vi "Main.vi"() -> ()   [LabVIEW 2019]
doc: "This template is for the Queued Message Handler design pattern.\n\nThe Event Handling Loop generates messages based on user interface actions.\n\nThe Message Handling Loop processes messages generated by the Event Handling Loop, or by other messages. The messages are string values, so new messages can be added easily to the Message Cases case structure in the Message Handling Loop. Each message cluster can also provide an optional value for Message Data, which is a variant that can be converted to whatever message-specific data is required."
uses:
  controls/UI Data.ctl
  controls/wavedump Data.ctl
  support/Message Queue/Enqueue Message (Single).vi
  <vilib>/Utility/error.llb/Error Cluster From Error Code.vi
  <vilib>/ErrorRing/Error Ring.xnode
  support/Message Queue/Message Queue.lvlib
  support/User Event - Stop/User Event - Stop.lvlib
panel:
  in  "power":bool
  in  "Off":bool
  in  "Tab Control":enum32{"Control", "Wavedump Output", "README"}(tab)
  in  "Gain":bool
  in  "HV Channel":string[](array[string])
  in  "DAQ Channel":string[](array[string])
  in  "PMT":string[](array[string])
  in  "Test":string(combo)
  in  "Run Time (s)":string
  in  "wavedump":bool
  in  "Run Number":string
  out "bash written":bool
  out "files cleared":bool
  out "wavedump finsihed":bool
  out "Power On":bool
  out "HV Monitor":T1={"Volt Monitor"=[["Ch", "ISet", "VSet", "VMon", "SWVMax", "IMon", "RUp", "RDwn", "Status\nV6534PA"], ["0", "200.000uA", "1500.000V", "1.200V", "2000V", "0.000uA", "100Vps", "250Vps", "OFF,\nV6534PA"], ["1", "200.000uA", "1820.000V", "0.000V", "2000V", "0.000uA", "100Vps", "250Vps", "OFF,\nV6534PA"], ["2", "200.000uA", "1380.000V", "0.000V", "2000V", "0.000uA", "100Vps", "250Vps", "OFF,\nV6534PA"], ["3", "200.000uA", "1280.000V", "1.200V", "2000V", "0.000uA", "100Vps", "250Vps", "OFF,\nV6534PA"], ["4", "200.000uA", "1320.000V", "0.000V", "2000V", "0.000uA", "100Vps", "250Vps", "OFF,\nV6534PA"], ["5", "0.000uA", "0.000V", "0.000V", "2000V", "0.000uA", "100Vps", "250Vps", "OFF,\nV6534PB"], ["0", "0.000uA", "0.000V", "1.500V", "2000V", "0.000uA", "100Vps", "250Vps", "OFF,\nV6534PB"], ["1", "0.000uA", "0.000V", "0.000V", "2000V", "0.000uA", "100Vps", "250Vps", "OFF,\nV6534PB"], ["2", "0.000uA", "0.000V", "0.000V", "2000V", "0.000uA", "100Vps", "250Vps", "OFF,\nV6534PB"], ["3", "0.000uA", "0.000V", "1.400V", "2000V", "0.000uA", "100Vps", "250Vps", "OFF,\nV6534PB"], ["4", "0.000uA", "0.000V", "0.000V", "2000V", "0.000uA", "100Vps", "250Vps", "OFF,\nV6534PB"], ["5", "0.000uA", "0.000V", "0.000V", "2000V", "0.000uA", "100Vps", "250Vps", "OFF,\nV6534PC"], ["0", "0.000uA", "0.000V", "1.400V", "2000V", "0.000uA", "100Vps", "250Vps", "OFF,\nV6534PC"], ["1", "0.000uA", "0.000V", "0.100V", "2000V", "0.000uA", "100Vps", "250Vps", "OFF,\nV6534PC"], ["2", "0.000uA", "0.000V", "0.000V", "2000V", "0.000uA", "100Vps", "250Vps", "OFF,\nV6534PC"], ["3", "0.000uA", "0.000V", "1.300V", "2000V", "0.000uA", "100Vps", "250Vps", "OFF,\nV6534PC"], ["4", "0.000uA", "0.000V", "0.300V", "2000V", "0.000uA", "100Vps", "250Vps", "OFF,\nV6534PC"], ["5", "0.000uA", "0.000V", "0.000V", "2000V", "0.000uA", "100Vps", "250Vps", "OFF,"]], "Power"=[FALSE, FALSE, FALSE, FALSE, FALSE, FALSE, FALSE, FALSE, FALSE, FALSE, FALSE, FALSE, FALSE, FALSE, FALSE, FALSE, FALSE, FALSE], "Rampup"=[FALSE, FALSE, FALSE, FALSE, FALSE, FALSE, FALSE, FALSE, FALSE, FALSE, FALSE, FALSE, FALSE, FALSE, FALSE, FALSE, FALSE, FALSE], "Rampdown"=[FALSE, FALSE, FALSE, FALSE, FALSE, FALSE, FALSE, FALSE, FALSE, FALSE, FALSE, FALSE, FALSE, FALSE, FALSE, FALSE, FALSE, FALSE], "Channel Errors"=["            \n", "            \n", "            \n", "            \n", "            \n", "            \n", "            \n", "            \n", "            \n", "            \n", "            \n", "            \n", "            \n", "            \n", "            \n", "            \n", "            \n", "            "], "Errors:\nMonitor       Status"=["Err: 0\nBoard", "Err: 0\n"]}
  in  "Channel                            Voltage (V)                      Current Max (uA)":string[][](array[string])=[["0", "0", "0", "Off"], ["1", "0", "0", "Off"], ["2", "0", "0", "Off"], ["3", "0", "0", "Off"], ["4", "0", "0", "Off"], ["5", "0", "0", "Off"], ["6", "0", "0", "Off"], ["7", "0", "0", "Off"], ["8", "0", "0", "Off"], ["9", "0", "0", "Off"], ["10", "0", "0", "Off"], ["11", "0", "0", "Off"], ["12", "0", "0", "Off"], ["13", "0", "0", "Off"], ["14", "0", "0", "Off"], ["15", "0", "0", "Off"], ["16", "0", "0", "Off"], ["17", "0", "0", "Off"]]
  in  "Power":bool[](array[boolean])=[FALSE, FALSE, FALSE, FALSE, FALSE, FALSE, FALSE, FALSE, FALSE, FALSE, FALSE, FALSE, FALSE, FALSE, FALSE, FALSE, FALSE, FALSE]
  in  "Max Voltage (V)":string="2000"
  in  "Ramp Up/Down":enum16{"Ramp Down", "Ramp Up"}(ring)=enum."Ramp Up"
  in  "Ramp Rate (V/s)":string="100"
  in  "ISet":bool
  in  "VSet":bool
  in  "Ramp":bool
  in  "VMax":bool
  out "HV Step":i32
  in  "Folder name":string
  out "Event Build Error":bool
  out "Over Temperature":bool
  out "Error":string="\n"
  out "Wavedump Output":string
  out "Test Control Readout":string="PMT Test Control"
  out "HV Control Readout":string="PMT Test Control"
  in  "Exit":bool
  # "Only the \"Exit\" button will work during a test run. Please wait for the test to finish or press \"Exit\" to turn the HV off and quit the program."
  # "Test control tab:\n\nThe Test Control tab contains controls needed to run PMT testing.\n\n1) Input PMT number, the digitiser channel it is plugged into and the HV channel it is plugged into.\n2) Select the test type, time to run test for and run number (default: 0) \n3) Press \"Run\" button\n\nWavedump terminal output will be shown in the output box inside the \"Wavedump Output\" tab upon run completion.\n\nThis requires the make file in the PMT_Testing directory to be run to compile the necessary software.\n\nThe HV settings, such as voltage, ramp rates and maximum current need to be set in the HV Control tab prior to running a test. The HV Monitor table will show the current state of the HV channels. The Test Control Tab will only power on the appropriate channels for the necessary time, not set the voltages to run at.\n\nThe Wavedump config file needs to be appropropriately setup prior to running this test.\n\nFiles will be moved to a date stamped folder one up from the PMT_Testing directory. This date stamped folder will contain time stamped folders for each run, which will in turn contain the PMT folders and their test files. \n\nHV Control tab:\n\nThis tab contains controls for the high voltage which can be used to set the parameters for testing or individually control the high voltage output of each channel.\n\nTo set voltages, input the desired values in volts into the \"Voltage\" column and then press the \"Voltage\" button to apply these settings.\n\nTo set a maximum current limit, enter the desired limits in microamps into the \"Max Current\" column and then press the \"Current\" button.\n\nTo set the maximum voltage (for all channels), enter the desired maximum voltage in volts into the \"Max Voltage\" box and then press the \"Max Voltage\" button.\n\nTo set the ramp rates for the voltage (all channels), enter the desired value in volts per second into the \"Ramp Rate\" box, select ramp up or ramp down and then press the \"Ramp\" button.\n\nTo turn channels on, press the power buttons for the desired channels in the array besides the table. Press the \"Power\" button at the top of the page to apply these settings. The chosen channels should switch on.\n\nTo turn the channels off, press the power buttons for the desired channels again to deselect them and then press the \"Power\" button at the top of the table. To turn all channels off at once, press the \"Off\" button at the top of the page.\n\nExit:\n\nTo turn all channels off and exit the application, press the \"Exit\" button at the top of the page.\n\nWhilst a test is running, only the \"Exit\" button will work until the test is done. If you need to cancel a test, press the \"Exit\" button and reopen the application.\n\nHV and Full Test readouts:\n\nThe HV and Full Test readouts at the top of the page will display the last command run in the relevant section."
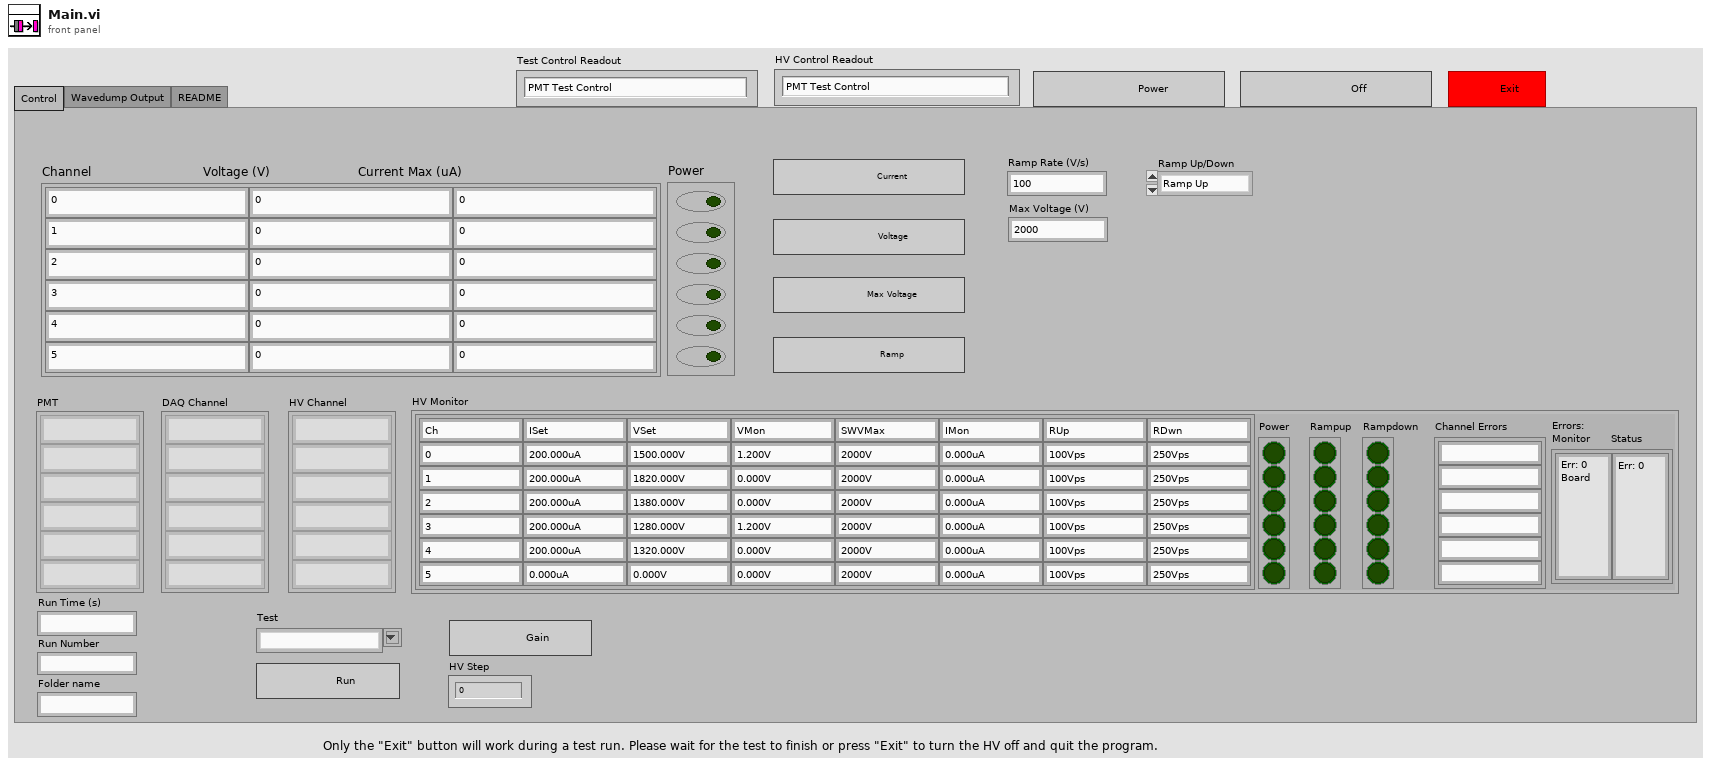
[diagram p1: front panel]
types:
  T1 = cluster{"Volt Monitor":string[][], "Power":bool[], "Rampup":bool[], "Rampdown":bool[], "Channel Errors":string[], "Errors:\nMonitor       Status":string[]}
  T2 = typedef "wavedump Data.ctl" = cluster{"String":string, "wavedump Ref":refnum<vi>, "Off Ref":refnum<vi>, "Data Display Ref":refnum<vi>, "Exit Button Ref":refnum<vi>}
  T3 = typedef "UI Data.ctl" = cluster{"String":string, "power Ref":refnum<vi>, "Off Ref":refnum<vi>, "Data Display Ref":refnum<vi>, "Exit Button Ref":refnum<vi>, "VSet Ref":refnum<vi>, "VMax Ref":refnum<vi>, "ISet Ref":refnum<vi>, "Ramp Ref":refnum<vi>}
  T4 = cluster{"Volt Monitor":string[][], "Power":bool[], "Rampup":bool[], "Rampdown":bool[], "Channel Errors":string[], "Errors:\nMonitor                Status":string[]}
  T5 = typedef "Message Queue.lvlib/All Message Queues.ctl" = cluster{"UI":refnum<queue>, "wavedump":refnum<queue>}
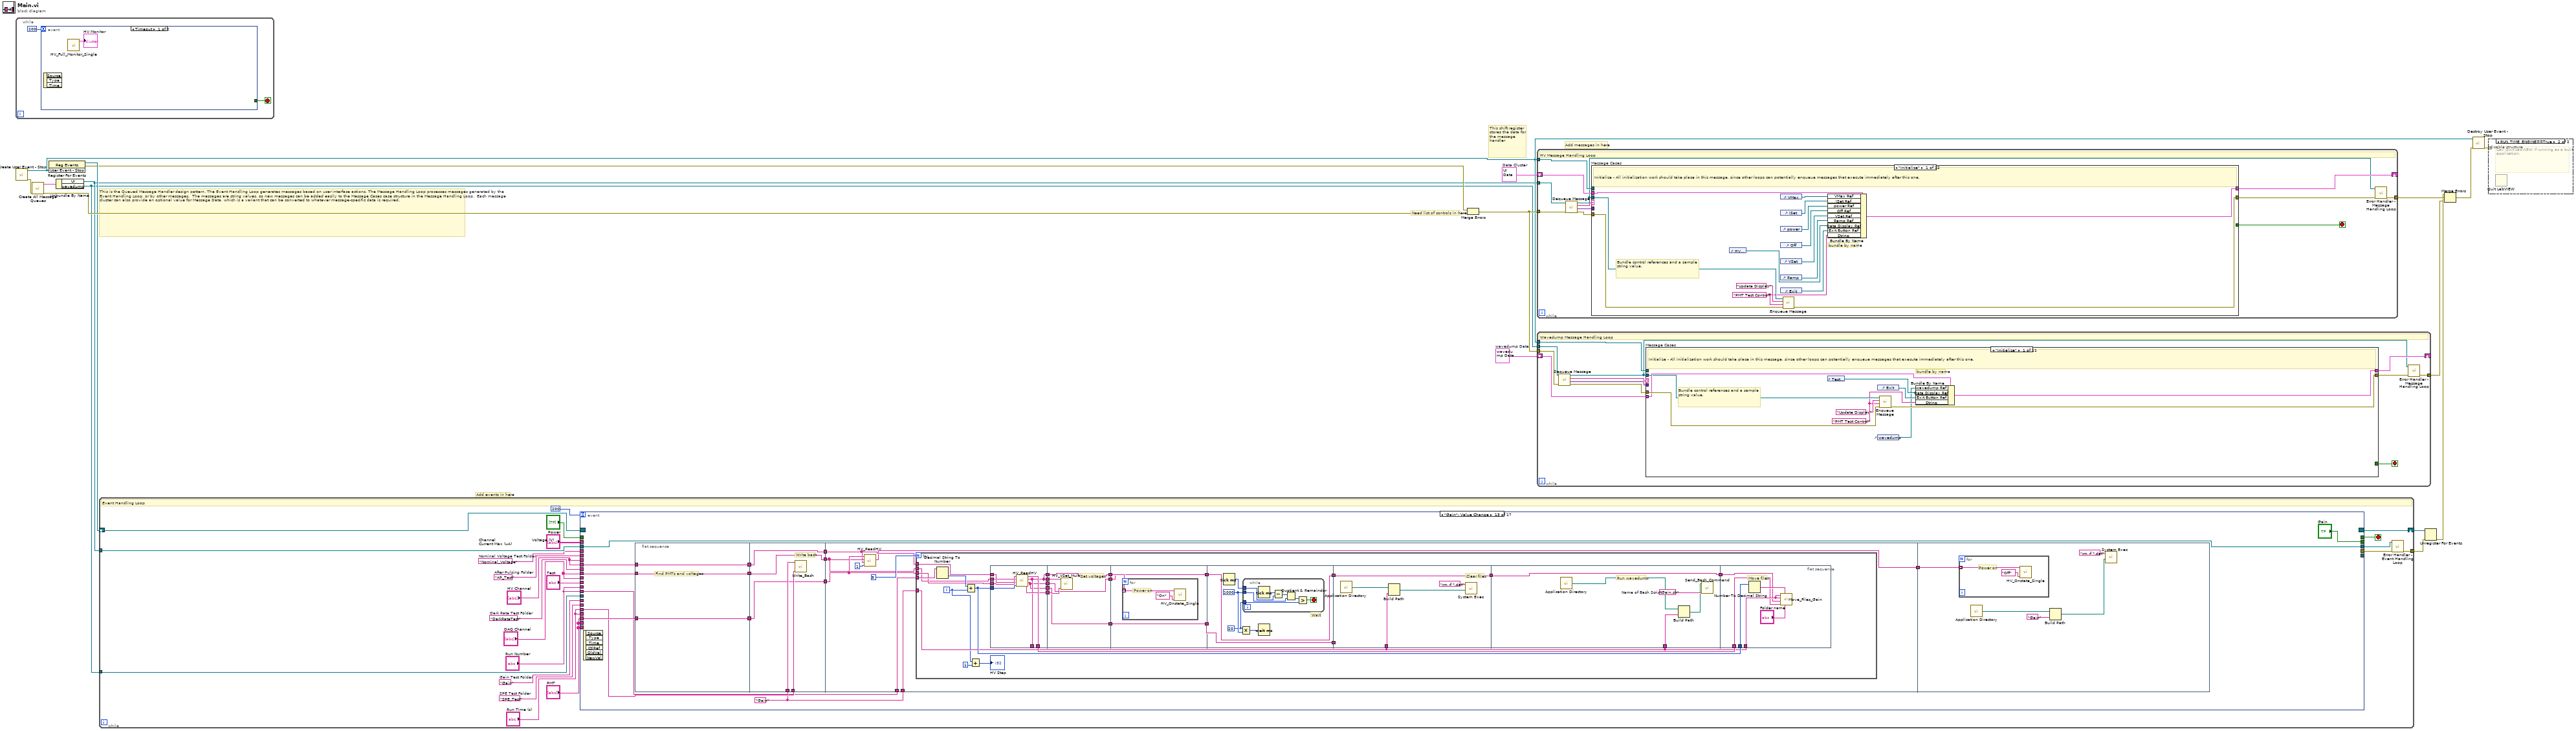
[diagram p0: block diagram]
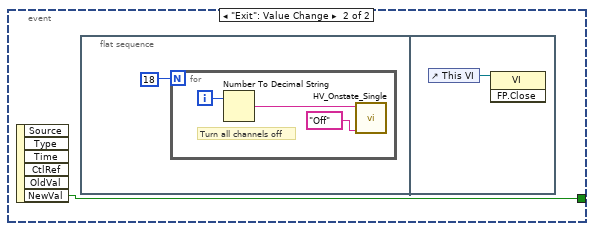
[diagram p2: hidden frame]
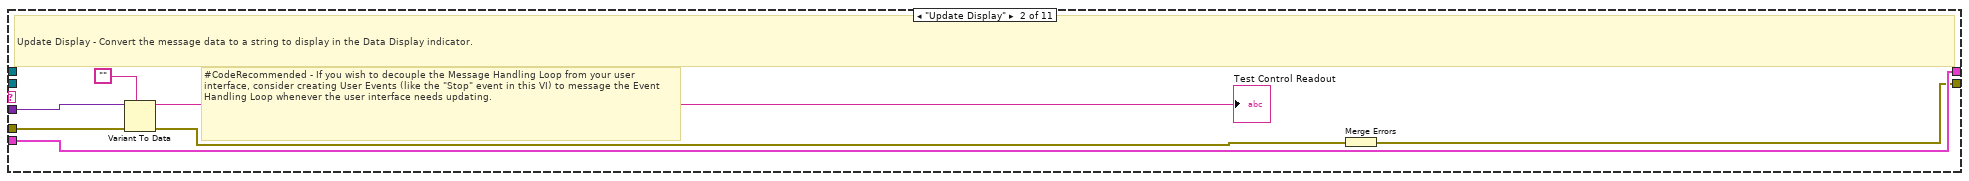
[diagram p3: hidden frame]
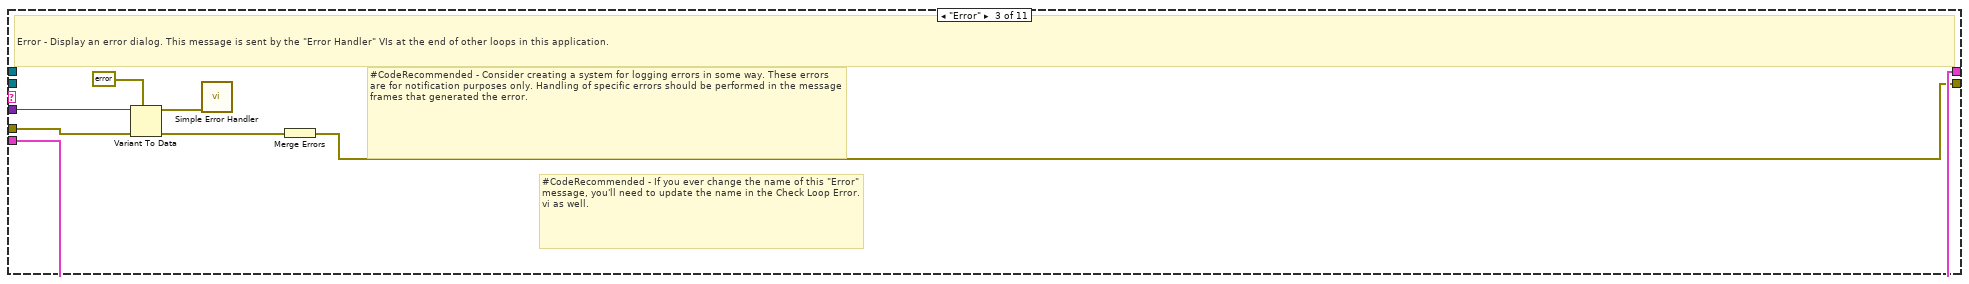
[diagram p4: hidden frame]
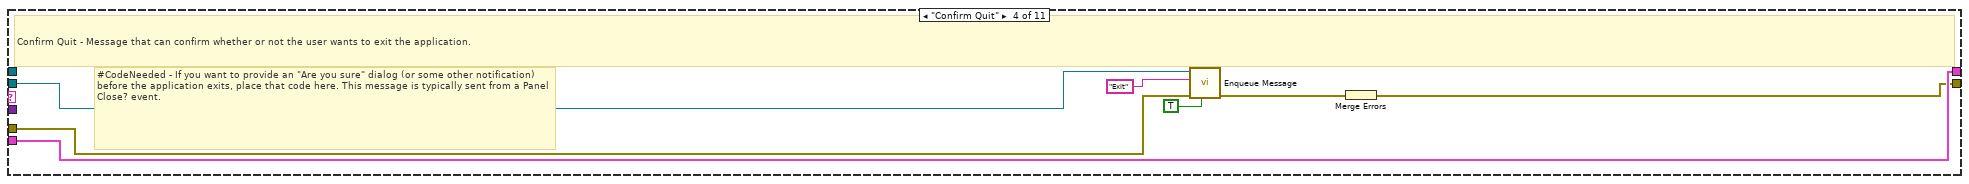
[diagram p5: hidden frame]
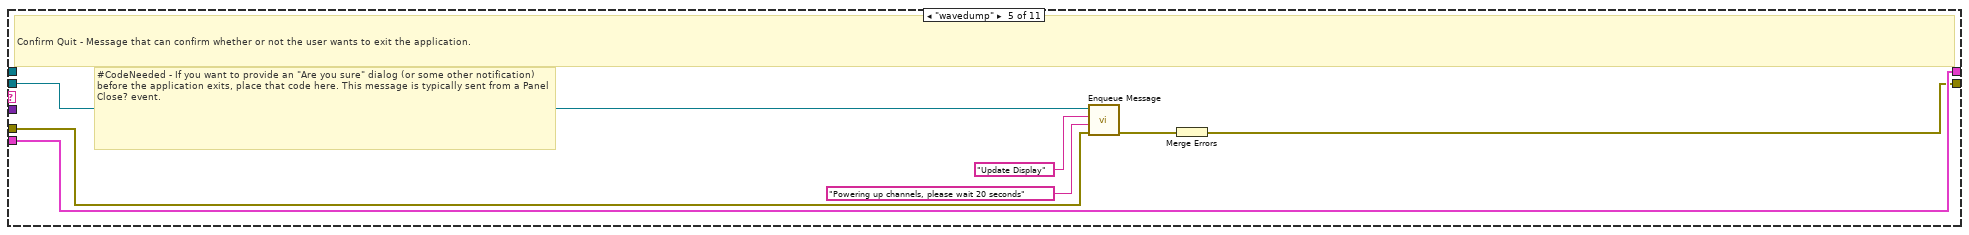
[diagram p6: hidden frame]
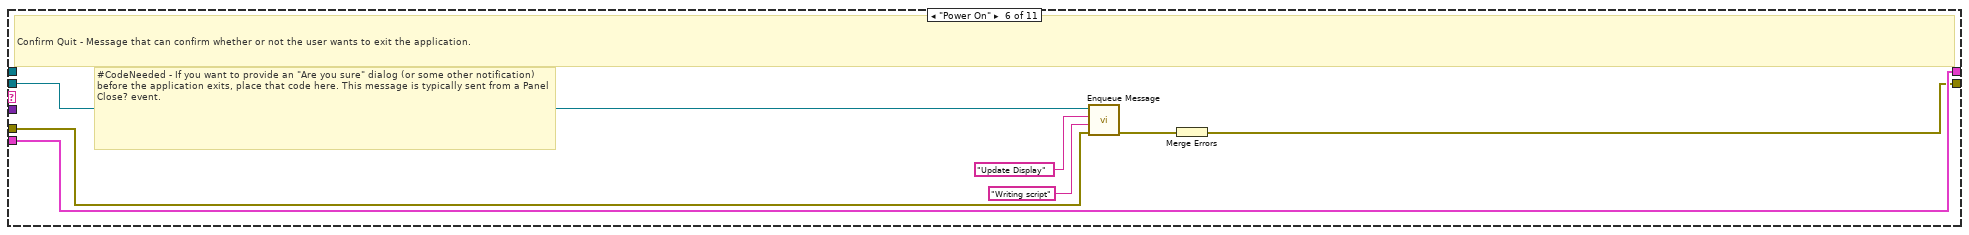
[diagram p7: hidden frame]
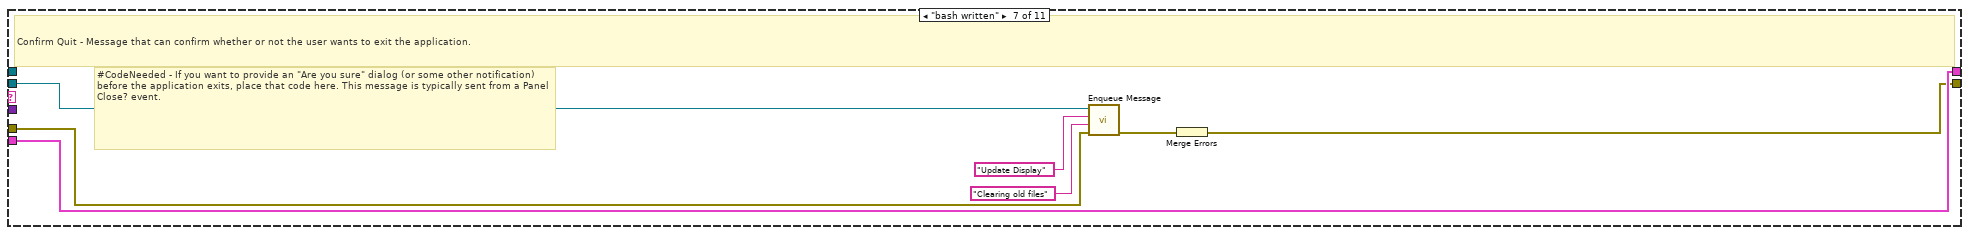
[diagram p8: hidden frame]
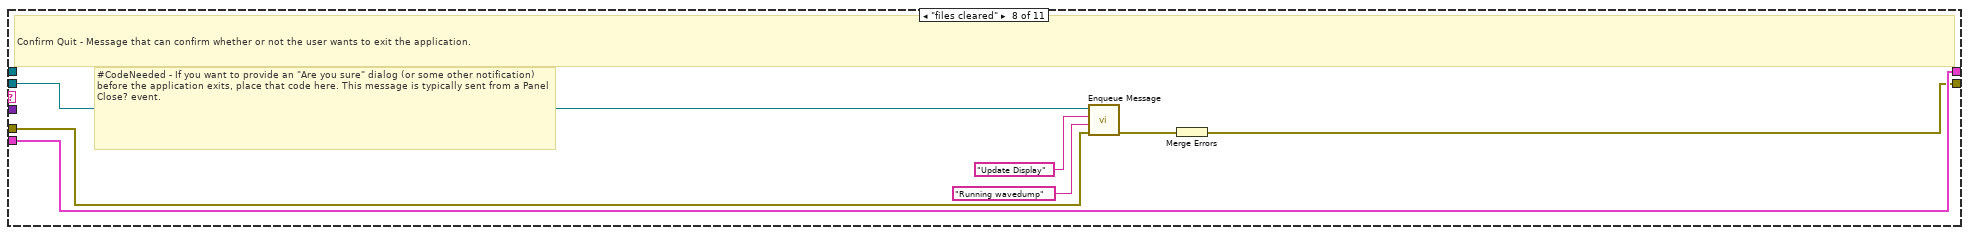
[diagram p9: hidden frame]
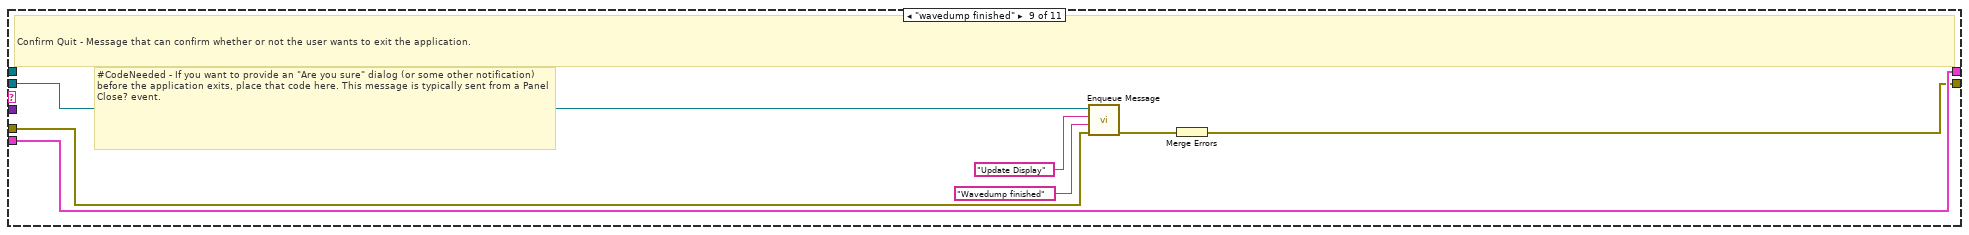
[diagram p10: hidden frame]
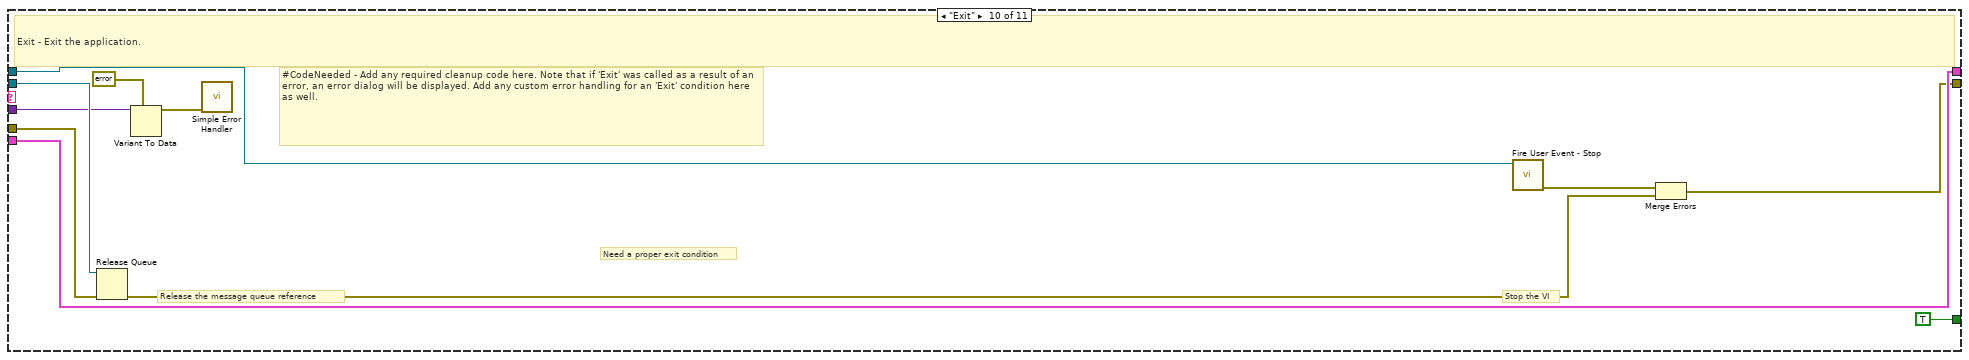
[diagram p11: hidden frame]
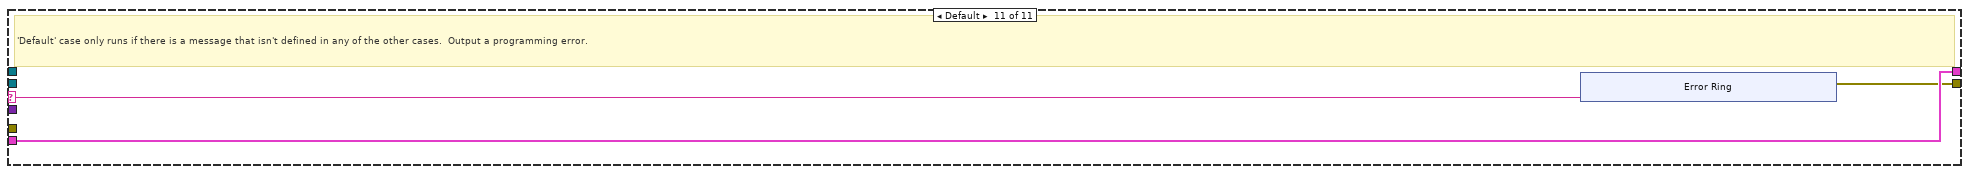
[diagram p12: hidden frame]
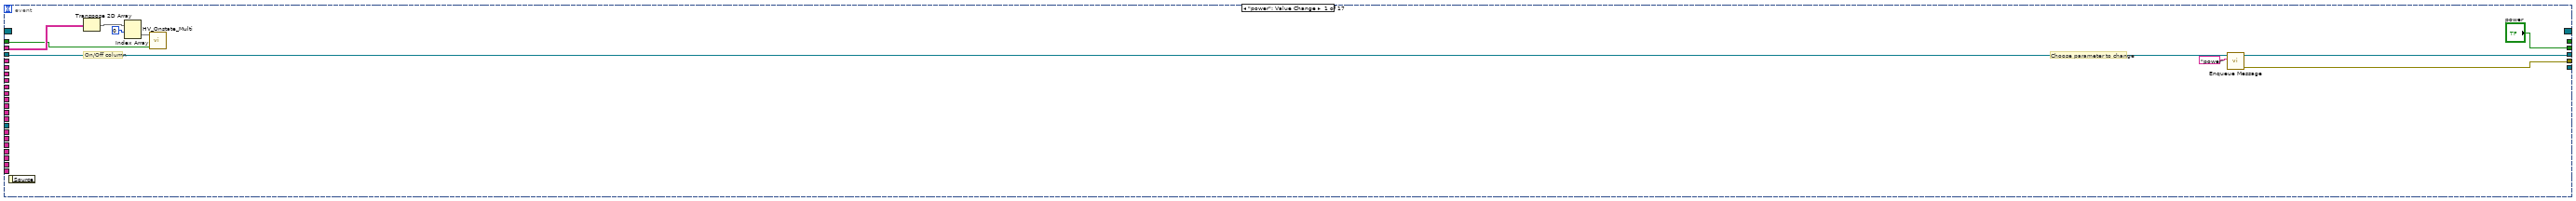
[diagram p14: hidden frame]
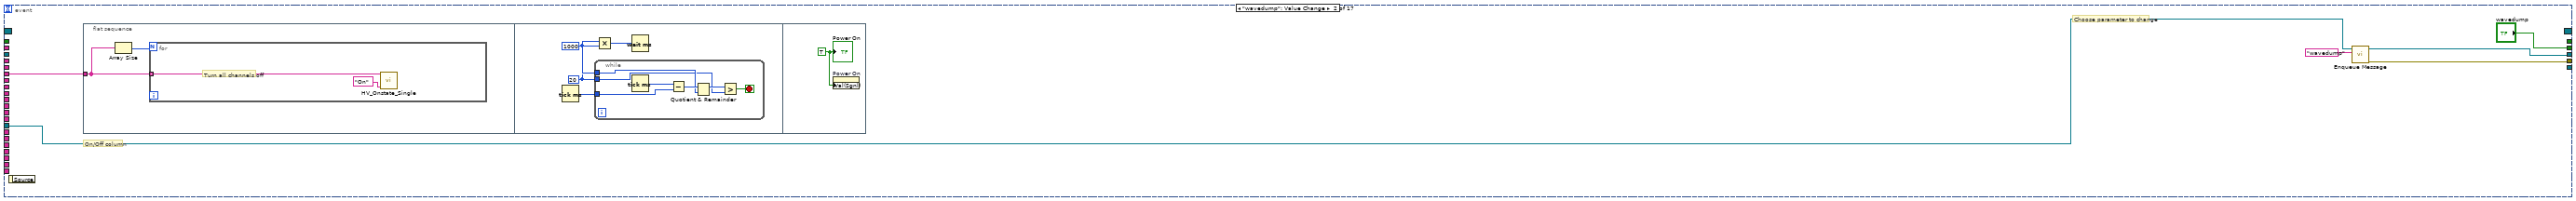
[diagram p15: hidden frame]
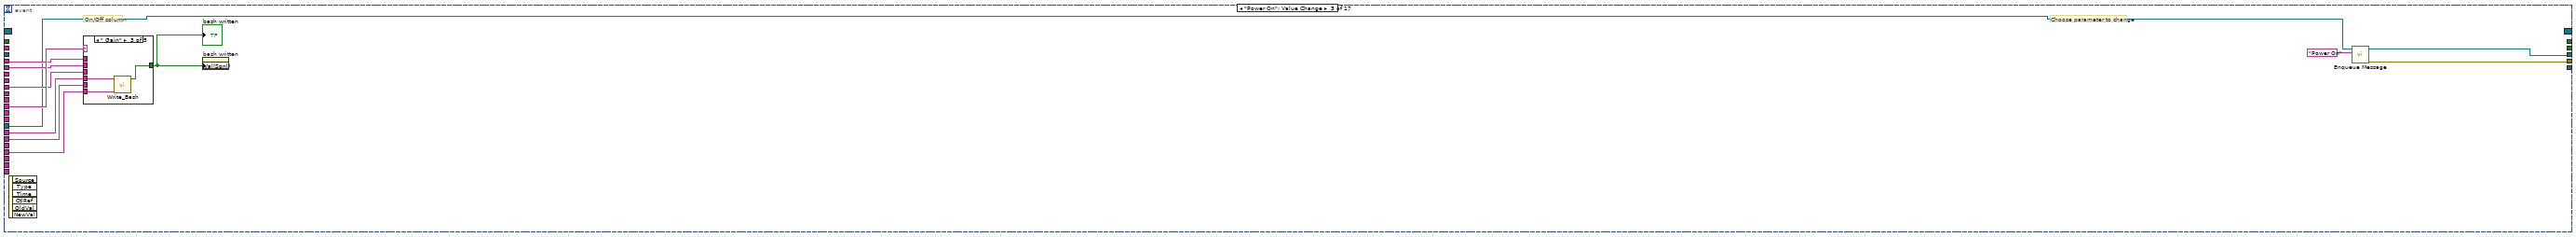
[diagram p16: hidden frame]
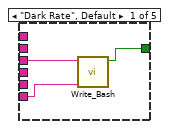
[diagram p17: hidden frame]
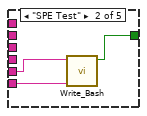
[diagram p18: hidden frame]
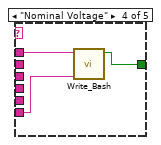
[diagram p19: hidden frame]
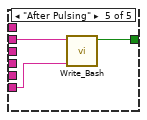
[diagram p20: hidden frame]
diagram:
  w2 = T2 {"String"="", "wavedump Ref"=refnum, "Off Ref"=refnum, "Data Display Ref"=refnum, "Exit Button Ref"=refnum}  # wavedump Data
  w3 = T3 {"String"="", "power Ref"=refnum, "Off Ref"=refnum, "Data Display Ref"=refnum, "Exit Button Ref"=refnum, "VSet Ref"=refnum, "VMax Ref"=refnum, "ISet Ref"=refnum, "Ramp Ref"=refnum}  # Data Cluster
  # "Need list of controls in here"
  # "Add messages in here"
  # "Add events in here"
  # "This is the Queued Message Handler design pattern. The Event Handling Loop generates messages based on user interface actions. The Message Handling Loop processes messages generated by the Event Handling Loop, or by other messages.  The messages are string values, so new messages can be added easily to the Message Cases case structure in the Message Handling Loop.  Each message cluster can also provide an optional value for Message Data, which is a variant that can be converted to whatever message-specific data is required."
  # "This shift register stores the data for the message handler"
  n1 = while {
    stop <- w19 stop-if-true
    n2 = event shown="[0] Timeout" {
      selector: _ -> [_ _]
      dyn-events: _ -> [_ _]
      timeout: 200 -> [_ _]
      tunnel: [_ w22] -> w19
      event Timeout {
        n3 = event-data() -> ()  [unwired: 1 in, 3 out]
        n4 = call "HV_Full_Monitor_Single.vi"() -> ("Monitor Cluster"=→"HV Monitor":T4)  [unwired: 11 in]
      }
      event "Exit": Value Change {
        n5 = event-data() -> ("NewVal"=w22:bool)  [unwired: 1 in, 5 out]
        n6 = flat-sequence {
          frame #0 {
            n7 = for {
              N: 18 -> [_]
              i -> [w25]
              # "Turn all channels off"
              n8 = Number To Decimal String(number=w25) -> (decimal integer string=w26:string)  [unwired: 1 in]
              n9 = call "HV_Onstate_Single.vi"("On/Off"="Off", "Channel"=w26) -> ()  [unwired: 9 in, 1 out]
            }
          }
          frame #1 {
            n10 = control-ref of="This VI"() -> (w27:refnum<vi>)
            n11 = invoke class="VI" method="FP.Close"(reference=w27) -> ()  [unwired: 2 in, 3 out]
          }
        }
      }
    }
  }
  n12 = call "Create User Event - Stop.vi"() -> ("error out"=w15:errorcluster, "User Event - Stop"=w6:refnum<user-event>)  [unwired: 10 in]
  n13 = call "Create All Message Queues.vi"("error in (no error)"=w15) -> ("error out"=w18:errorcluster, "Message Queues out"=w17:T5)  [unwired: 9 in]
  n14 = register-events(w6) -> (reference out=w9:refnum<event-registration>, error out=w8:errorcluster)  [unwired: 2 in]
  n15 = Unbundle By Name(w17) -> ("UI"=w4:refnum<queue>, "wavedump"=w1:refnum<queue>)
  n16 = while {
    tunnel: w4 -> [w49]
    shift-right: [w47] -> w12
    shift-left: w9 -> [w48]
    tunnel: [w43] -> w10
    tunnel: w1 -> [w40]
    stop <- w45 stop-if-true
    w38 = "SPE_Test"  # SPE Test Folder
    w35 = "AP_Test"  # After Pulsing Folder
    w34 = "DarkRateTest"  # Dark Rate Test Folder
    w36 = "Nominal_Voltage"  # Nominal Voltage Test Folder
    w37 = "Gain"  # Gain Test Folder
    # "Event Handling Loop"
    n17 = event shown="[12] \"Gain\": Value Change" {
      selector: w48 -> [_ _ _ _ _ _ _ _ _ _ _ _ _ _ _ _ _]
      dyn-events: [_ _ _ _ _ _ _ _ _ _ _ _ _ _ _ _ _] -> w47
      timeout: 200 -> [_ _ _ _ _ _ _ _ _ _ _ _ _ _ _ _ _]
      tunnel: [_ _ _ _ _ _ _ _ _ _ _ _ _ _ _ _ TRUE ("Discard?")] -> w45
      tunnel: w49 -> [w55 _ _ _ _ _ w239 w243 w255 w267 w273 w282 w302 w402 w405 w414 w421]
      tunnel: [w52 w63 w91 w118 w149 w208 _ w240 w252 w264 w270 w281 _ w401 _ w413 _] -> w46
      tunnel: [w54 w65 w93 w120 w151 w210 w239 w242 w254 w266 w272 w283 w302 w400 w405 w412 w421] -> w44
      tunnel: ["power" "wavedump" _ _ _ _ _ "ISet" "VSet" "VMax" "Ramp" "Off" "Gain" _ _ _ _] -> _
      tunnel: "Channel                            Voltage (V)                      Current Max (uA)" -> [w51 _ _ _ _ _ _ w244 w256 _ _ _ _ _ _ _ _]
      tunnel: w40 -> [_ w61 w83 w117 w148 w207 _ _ _ _ _ _ _ _ _ _ w418]
      tunnel: "Test" -> [_ _ w90 w116 w142 w206 _ _ _ _ _ _ _ _ _ _ _]
      tunnel: w38 -> [_ _ w89 w110 w137 w199 _ _ _ _ _ _ _ _ _ _ _]
      tunnel: "Run Time (s)" -> [_ _ w88 _ _ _ _ _ _ _ _ _ _ _ _ _ _]
      tunnel: w37 -> [_ _ w87 w113 w141 w198 _ _ _ _ _ _ _ _ _ _ _]
      tunnel: w36 -> [_ _ w86 w112 w140 w202 _ _ _ _ _ _ _ _ _ _ _]
      tunnel: w35 -> [_ _ w85 w114 w139 w201 _ _ _ _ _ _ _ _ _ _ _]
      tunnel: w34 -> [_ _ w84 w111 w138 w200 _ _ _ _ _ _ _ _ _ _ _]
      tunnel: "DAQ Channel" -> [_ _ _ w115 _ w204 _ _ _ _ _ _ _ _ _ _ _]
      tunnel: "PMT" -> [_ _ _ _ _ w205 _ _ _ _ _ _ _ _ _ _ _]
      tunnel: "Run Number" -> [_ _ _ _ _ w203 _ _ _ _ _ _ _ _ _ _ _]
      tunnel: [_ _ _ _ _ _ _ _ _ _ _ _ _ _ _ _ w418] -> _
      tunnel: "HV Channel" -> [_ w60 _ _ _ _ _ _ _ _ _ _ _ _ _ _ _]
      tunnel: "Power" -> [w50 _ _ _ _ _ _ _ _ _ _ _ _ _ _ _ _]
      tunnel: "PMT" -> [_ _ _ _ _ _ _ _ _ _ _ _ _ _ _ _ _]
      tunnel: "PMT" -> [_ _ _ _ _ _ _ _ _ _ _ _ w300 _ _ _ _]
      tunnel: "DAQ Channel" -> [_ _ _ _ _ _ _ _ _ _ _ _ w299 _ _ _ _]
      tunnel: "HV Channel" -> [_ _ _ _ _ _ _ _ _ _ _ _ w298 _ _ _ _]
      tunnel: "Run Time (s)" -> [_ _ _ _ _ _ _ _ _ _ _ _ w297 _ _ _ _]
      tunnel: "Run Number" -> [_ _ _ _ _ _ _ _ _ _ _ _ w295 _ _ _ _]
      event "power": Value Change {
        # "On/Off column"
        # "Choose parameter to change"
        n18 = event-data() -> ()  [unwired: 1 in, 1 out]
        n19 = Transpose 2D Array(2D array=w51) -> (transposed array=w58:string[][])
        n20 = Index Array(array=w58, index (row)=0) -> (element=w57:string[])  [unwired: 1 in]
        n21 = call "HV_Onstate_Multi.vi"("Power"=w50, "Channel"=w57) -> ()  [unwired: 9 in, 1 out]
        n22 = call-poly "Enqueue Message.vi"("Message"="power", "Message Queue"=w55) -> ("error out"=w52:errorcluster, "dup Message Queue"=w54:refnum<queue>)  [unwired: 8 in]
      }
      event "wavedump": Value Change {
        # "On/Off column"
        # "Choose parameter to change"
        n23 = event-data() -> ()  [unwired: 1 in, 1 out]
        n24 = flat-sequence {
          tunnel: w60 -> [w66]
          frame #0 {
            n25 = Array Size(array=w66) -> (size(s)=w67:i32)
            n26 = for {
              N: w67 -> [_]
              tunnel: w66 -> [w68] mode=indexing
              # "Turn all channels off"
              n27 = call "HV_Onstate_Single.vi"("On/Off"="On", "Channel"=w68) -> ()  [unwired: 9 in, 1 out]
            }
          }
          frame #1 {
            w71 = 1000 ("y")
            w70 = 20
            n28 = Tick Count (ms)() -> (millisecond timer value=w72:u32)
            n29 = while {
              tunnel: w72 -> [w79]
              tunnel: w71 -> [w77]
              tunnel: w70 -> [w75]
              stop <- w74 stop-if-true
              n30 = Tick Count (ms)() -> (millisecond timer value=w80:u32)
              n31 = Subtract(x=w80, y=w79) -> (x-y=w78:u32)
              n32 = Quotient & Remainder(x=w78, y=w77) -> (x-y*floor(x/y)=w76:u32)  [unwired: 1 out]
              n33 = Greater?(x=w76, y=w75) -> (0:w74:bool)
            }
            n34 = Multiply(x=w70, y=w71) -> (x*y=w73:i32)
            n35 = Wait (ms)(milliseconds to wait=w73) -> ()  [unwired: 1 out]
          }
          frame #2 {
            w81 = TRUE
            n36 = property on="Power On" class="Bool (strict)"("Val(Sgnl)"=w81) -> ()  [unwired: 2 in, 2 out]
            "Power On" <- w81
          }
        }
        n37 = call-poly "Enqueue Message.vi"("Message"="wavedump", "Message Queue"=w61) -> ("error out"=w63:errorcluster, "dup Message Queue"=w65:refnum<queue>)  [unwired: 8 in]
      }
      event "Power On": Value Change {
        # "On/Off column"
        # "Choose parameter to change"
        n38 = event-data() -> ()  [unwired: 1 in, 6 out]
        n39 = case shown="\" Gain\"" w90 {
          tunnel: w88 -> [w96 w99 w101 w104 w107]
          tunnel: w84 -> [w95 _ _ _ _]
          tunnel: w87 -> [_ _ w102 _ _]
          tunnel: w86 -> [_ _ _ w105 _]
          tunnel: w85 -> [_ _ _ _ w108]
          tunnel: w89 -> [_ w98 _ _ _]
          tunnel: [w94 w97 w100 w103 w106] -> w82
          frame "Dark Rate", Default {
            n40 = call "Write_Bash.vi"("Time"=w96, "Test"=w95) -> ("bash written"=w94:bool)  [unwired: 9 in]
          }
          frame "SPE Test" {
            n41 = call "Write_Bash.vi"("Time"=w99, "Test"=w98) -> ("bash written"=w97:bool)  [unwired: 9 in]
          }
          frame " Gain" {
            n42 = call "Write_Bash.vi"("Time"=w101, "Test"=w102) -> ("bash written"=w100:bool)  [unwired: 9 in]
          }
          frame "Nominal Voltage" {
            n43 = call "Write_Bash.vi"("Time"=w104, "Test"=w105) -> ("bash written"=w103:bool)  [unwired: 9 in]
          }
          frame "After Pulsing" {
            n44 = call "Write_Bash.vi"("Time"=w107, "Test"=w108) -> ("bash written"=w106:bool)  [unwired: 9 in]
          }
        }
        "bash written" <- w82
        n45 = property on="bash written" class="Bool (strict)"("Val(Sgnl)"=w82) -> ()  [unwired: 2 in, 2 out]
        n46 = call-poly "Enqueue Message.vi"("Message"="Power On", "Message Queue"=w83) -> ("error out"=w91:errorcluster, "dup Message Queue"=w93:refnum<queue>)  [unwired: 8 in]
      }
      event "bash written": Value Change {
        # "Choose parameter to change"
        n47 = event-data() -> ()  [unwired: 1 in, 6 out]
        n48 = case shown="\"Gain\", Default" w116 {
          tunnel: w115 -> [w123 w126 w129 w132 w135]
          tunnel: w111 -> [_ _ _ w131 _]
          tunnel: w110 -> [_ _ _ _ w134]
          tunnel: w114 -> [w122 _ _ _ _]
          tunnel: w113 -> [_ w125 _ _ _]
          tunnel: w112 -> [_ _ w128 _ _]
          tunnel: [w121 w124 w127 w130 w133] -> w109
          frame "After Pulsing" {
            n49 = call "Clear_Old_Files.vi"("Bash Script Folder Name"=w122, "Channel"=w123) -> ("files cleared"=w121:bool)  [unwired: 8 in, 1 out]
          }
          frame "Gain", Default {
            n50 = call "Clear_Old_Files.vi"("Bash Script Folder Name"=w125, "Channel"=w126) -> ("files cleared"=w124:bool)  [unwired: 8 in, 1 out]
          }
          frame "Nominal Voltage" {
            n51 = call "Clear_Old_Files.vi"("Bash Script Folder Name"=w128, "Channel"=w129) -> ("files cleared"=w127:bool)  [unwired: 8 in, 1 out]
          }
          frame "Dark Rate" {
            n52 = call "Clear_Old_Files.vi"("Bash Script Folder Name"=w131, "Channel"=w132) -> ("files cleared"=w130:bool)  [unwired: 8 in, 1 out]
          }
          frame "SPE Test" {
            n53 = call "Clear_Old_Files.vi"("Bash Script Folder Name"=w134, "Channel"=w135) -> ("files cleared"=w133:bool)  [unwired: 8 in, 1 out]
          }
        }
        "files cleared" <- w109
        n54 = property on="files cleared" class="Bool (strict)"("Val(Sgnl)"=w109) -> ()  [unwired: 2 in, 2 out]
        n55 = call-poly "Enqueue Message.vi"("Message"="bash written", "Message Queue"=w117) -> ("error out"=w118:errorcluster, "dup Message Queue"=w120:refnum<queue>)  [unwired: 8 in]
      }
      event "files cleared": Value Change {
        # "Add config file input option"
        # "Choose parameter to change"
        n56 = event-data() -> ()  [unwired: 1 in, 6 out]
        n57 = call <vilib>:"Application Directory.vi"() -> ("Application Directory"=w147:path)
        n58 = case shown="\"Gain\", Default" w142 {
          tunnel: [w154 w163 w172 w181 w190] -> w143
          tunnel: [w155 w164 w173 w182 w191] -> w144
          tunnel: [w156 w165 w174 w183 w192] -> w145
          tunnel: [w157 w166 w175 w184 w193] -> w146
          tunnel: w147 -> [w158 w167 w176 w186 w194]
          tunnel: w141 -> [w153 _ _ _ _]
          tunnel: w137 -> [_ _ _ _ w189]
          tunnel: w138 -> [_ _ _ w180 _]
          tunnel: w139 -> [_ _ w171 _ _]
          tunnel: w140 -> [_ w162 _ _ _]
          tunnel: [w152 w161 w170 w179 w188] -> w136
          frame "Gain", Default {
            w160 = "Gain.sh"  # Name of Bash Script
            n59 = Build Path(base path=w158, name or relative path=w153) -> (appended path=w159:path)
            n60 = call "Send_Bash_Command.vi"("working directory"=w159, "Bash script"=w160) -> ("wavedump finsihed"=w152:bool, "Command Line Output"=w157:string, "Over Temperature"=w156:bool, "Event Build Error"=w155:bool, "Error"=w154:string)  [unwired: 4 in]
          }
          frame "Nominal Voltage" {
            w169 = "Nominal_Voltage.sh"  # Name of Bash Script
            n61 = Build Path(base path=w167, name or relative path=w162) -> (appended path=w168:path)
            n62 = call "Send_Bash_Command.vi"("working directory"=w168, "Bash script"=w169) -> ("wavedump finsihed"=w161:bool, "Command Line Output"=w166:string, "Over Temperature"=w165:bool, "Event Build Error"=w164:bool, "Error"=w163:string)  [unwired: 4 in]
          }
          frame "After Pulsing" {
            w178 = "AP_Test.sh"  # Name of Bash Script
            n63 = Build Path(base path=w176, name or relative path=w171) -> (appended path=w177:path)
            n64 = call "Send_Bash_Command.vi"("working directory"=w177, "Bash script"=w178) -> ("wavedump finsihed"=w170:bool, "Command Line Output"=w175:string, "Over Temperature"=w174:bool, "Event Build Error"=w173:bool, "Error"=w172:string)  [unwired: 4 in]
          }
          frame "Dark Rate" {
            w185 = "DarkRateTest.sh"  # Name of Bash Script
            n65 = Build Path(base path=w186, name or relative path=w180) -> (appended path=w187:path)
            n66 = call "Send_Bash_Command.vi"("working directory"=w187, "Bash script"=w185) -> ("wavedump finsihed"=w179:bool, "Command Line Output"=w184:string, "Over Temperature"=w183:bool, "Event Build Error"=w182:bool, "Error"=w181:string)  [unwired: 4 in]
          }
          frame "SPE Test" {
            w196 = "SPE_Test.sh"  # Name of Bash Script
            n67 = Build Path(base path=w194, name or relative path=w189) -> (appended path=w195:path)
            n68 = call "Send_Bash_Command.vi"("working directory"=w195, "Bash script"=w196) -> ("wavedump finsihed"=w188:bool, "Command Line Output"=w193:string, "Over Temperature"=w192:bool, "Event Build Error"=w191:bool, "Error"=w190:string)  [unwired: 4 in]
          }
        }
        "Wavedump Output" <- w146
        "Over Temperature" <- w145
        "Event Build Error" <- w144
        "Error" <- w143
        "wavedump finsihed" <- w136
        n69 = property on="wavedump finsihed" class="Bool (strict)"("Val(Sgnl)"=w136) -> ()  [unwired: 2 in, 2 out]
        n70 = call-poly "Enqueue Message.vi"("Message"="files cleared", "Message Queue"=w148) -> ("error out"=w149:errorcluster, "dup Message Queue"=w151:refnum<queue>)  [unwired: 8 in]
      }
      event "wavedump finsihed": Value Change {
        # "Choose parameter to change"
        n71 = event-data() -> ()  [unwired: 1 in, 6 out]
        n72 = case shown="\"Gain\", Default" w206 {
          tunnel: w205 -> [w217 w222 w227 w232 w237]
          tunnel: w203 -> [w216 w220 w225 w231 w236]
          tunnel: w204 -> [w215 w221 w226 w230 w235]
          tunnel: w198 -> [w214 _ _ _ _]
          tunnel: w199 -> [_ _ _ _ w234]
          tunnel: w200 -> [_ _ _ w229 _]
          tunnel: w201 -> [_ _ w224 _ _]
          tunnel: w202 -> [_ w219 _ _ _]
          frame "Gain", Default {
            w218 = "Gain"  # Name of Folder to Copy PMT File to
            n73 = call "Move_Files.vi"("Run"=w216, "PMTs"=w217, "Channel"=w215, "Folder Containing Bash Script"=w214, "Name of Folder to\nCopy PMT File to"=w218) -> ()  [unwired: 7 in]
          }
          frame "Nominal Voltage" {
            w223 = "Nominal_Voltage"  # Name of Folder to Copy PMT File to
            n74 = call "Move_Files.vi"("Run"=w220, "PMTs"=w222, "Channel"=w221, "Folder Containing Bash Script"=w219, "Name of Folder to\nCopy PMT File to"=w223) -> ()  [unwired: 7 in]
          }
          frame "After Pulsing" {
            w228 = "After_Pulsing"  # Name of Folder to Copy PMT File to
            n75 = call "Move_Files.vi"("Run"=w225, "PMTs"=w227, "Channel"=w226, "Folder Containing Bash Script"=w224, "Name of Folder to\nCopy PMT File to"=w228) -> ()  [unwired: 7 in]
          }
          frame "Dark Rate" {
            w233 = "DarkRate"  # Name of Folder to Copy PMT File to
            n76 = call "Move_Files.vi"("Run"=w231, "PMTs"=w232, "Channel"=w230, "Folder Containing Bash Script"=w229, "Name of Folder to\nCopy PMT File to"=w233) -> ()  [unwired: 7 in]
          }
          frame "SPE Test" {
            w238 = "SPE_Test"  # Name of Folder to Copy PMT File to
            n77 = call "Move_Files.vi"("Run"=w236, "PMTs"=w237, "Channel"=w235, "Folder Containing Bash Script"=w234, "Name of Folder to\nCopy PMT File to"=w238) -> ()  [unwired: 7 in]
          }
        }
        n78 = for {
          N: 18 -> [_]
          i -> [w212]
          # "Turn all channels off"
          n79 = Number To Decimal String(number=w212) -> (decimal integer string=w213:string)  [unwired: 1 in]
          n80 = call "HV_Onstate_Single.vi"("On/Off"="Off", "Channel"=w213) -> ()  [unwired: 9 in, 1 out]
        }
        n81 = call-poly "Enqueue Message.vi"("Message"="wavedump finished", "Message Queue"=w207) -> ("error out"=w208:errorcluster, "dup Message Queue"=w210:refnum<queue>)  [unwired: 8 in]
      }
      event Timeout {
        n82 = event-data() -> ()  [unwired: 1 in, 3 out]
      }
      event "ISet": Value Change {
        n83 = event-data() -> ()  [unwired: 1 in, 6 out]
        n84 = Transpose 2D Array(2D array=w244) -> (transposed array=w250:string[][])
        n85 = Transpose 2D Array(2D array=w244) -> (transposed array=w248:string[][])
        n86 = Index Array(array=w250, index (row)=0) -> (element=w247:string[])  [unwired: 1 in]
        n87 = Index Array(array=w248, index (row)=2) -> (element=w246:string[])  [unwired: 1 in]
        n88 = call "HV_ISet_Multi.vi"("Currents"=w246, "Channels"=w247) -> ()  [unwired: 9 in, 1 out]
        n89 = call-poly "Enqueue Message.vi"("Message"="ISet", "Message Queue"=w243) -> ("error out"=w240:errorcluster, "dup Message Queue"=w242:refnum<queue>)  [unwired: 8 in]
      }
      event "VSet": Value Change {
        # "Voltage column"
        # "Channels column"
        n90 = event-data() -> ()  [unwired: 1 in, 6 out]
        n91 = Transpose 2D Array(2D array=w256) -> (transposed array=w261:string[][])
        n92 = Transpose 2D Array(2D array=w256) -> (transposed array=w258:string[][])
        n93 = Index Array(array=w261, index (row)=0) -> (element=w260:string[])  [unwired: 1 in]
        n94 = Index Array(array=w258, index (row)=1) -> (element=w257:string[])  [unwired: 1 in]
        n95 = call "HV_VSet_Multi.vi"("Voltage"=w257, "Channel"=w260) -> ()  [unwired: 9 in, 1 out]
        n96 = call-poly "Enqueue Message.vi"("Message"="VSet", "Message Queue"=w255) -> ("error out"=w252:errorcluster, "dup Message Queue"=w254:refnum<queue>)  [unwired: 8 in]
      }
      event "VMax": Value Change {
        n97 = event-data() -> ()  [unwired: 1 in, 6 out]
        n98 = call "HV_SWVMaxSet.vi"("Max Voltage"="Max Voltage (V)") -> ()  [unwired: 10 in, 1 out]
        n99 = call-poly "Enqueue Message.vi"("Message"="VMax", "Message Queue"=w267) -> ("error out"=w264:errorcluster, "dup Message Queue"=w266:refnum<queue>)  [unwired: 8 in]
      }
      event "Ramp": Value Change {
        n100 = event-data() -> ()  [unwired: 1 in, 6 out]
        n101 = call "HV_Rampset.vi"("Ramp Up/Down"="Ramp Up/Down", "Ramp Rate"="Ramp Rate (V/s)") -> ()  [unwired: 9 in, 1 out]
        n102 = call-poly "Enqueue Message.vi"("Message"="Ramp", "Message Queue"=w273) -> ("error out"=w270:errorcluster, "dup Message Queue"=w272:refnum<queue>)  [unwired: 8 in]
      }
      event "Off": Value Change {
        w278 = 18
        n103 = event-data() -> ()  [unwired: 1 in, 6 out]
        n104 = for {
          N: w278 -> [_]
          i -> [w286]
          # "Turn all channels off"
          n105 = Number To Decimal String(number=w286) -> (decimal integer string=w287:string)  [unwired: 1 in]
          n106 = call "HV_Onstate_Single.vi"("On/Off"="Off", "Channel"=w287) -> ()  [unwired: 9 in, 1 out]
        }
        n107 = Initialize Array(FALSE, w278) -> (w277:bool[])
        n108 = local write "Power"(w277) -> ()
        n109 = call-poly "Enqueue Message.vi"("Message"="Off", "Message Queue"=w282) -> ("error out"=w281:errorcluster, "dup Message Queue"=w283:refnum<queue>)  [unwired: 8 in]
      }
      event "Gain": Value Change {
        w296 = "Gain" ("Test")
        n110 = event-data() -> ()  [unwired: 1 in, 6 out]
        n111 = flat-sequence {
          tunnel: w300 -> [w305]
          tunnel: w299 -> [w304]
          tunnel: w298 -> [w303]
          tunnel: [w305] -> w294
          tunnel: [w304] -> w292
          tunnel: [w303] -> w290
          tunnel: w297 -> [w310]
          tunnel: w296 -> [w309]
          tunnel: w294 -> [w308]
          tunnel: [w308] -> w293
          tunnel: w292 -> [w307]
          tunnel: [w307] -> w291
          tunnel: w290 -> [w306]
          tunnel: [w306] -> w289
          tunnel: w296 -> [w317]
          tunnel: w295 -> [w316]
          tunnel: w293 -> [w315]
          tunnel: w291 -> [w313]
          tunnel: w289 -> [w312]
          tunnel: [w311] -> w288
          tunnel: w288 -> [w395]
          frame #0 {
            # "Find PMTs and voltages"
          }
          frame #1 {
            # "Write bash"
            n112 = call "Write_Bash.vi"("Time"=w310, "Test"=w309) -> ()  [unwired: 9 in, 1 out]
          }
          frame #2 {
            n113 = call "HV_ReadHV.vi"("Run"=1, "HV Channel"=w312, "DAQ Channel"=w313, "PMT"=w315) -> ("HV Channel Out"=w311:string[])  [unwired: 4 in, 3 out]
            n114 = for {
              N: 5 -> [_]
              tunnel: w317 -> [w322]
              tunnel: w316 -> [w343]
              tunnel: w315 -> [w340]
              tunnel: w313 -> [w339]
              tunnel: w312 -> [w338]
              i -> [w320]
              n115 = Decimal String To Number(string=w343) -> (number=w342:i32)  [unwired: 2 in, 1 out]
              n116 = Add(x=w342, y=w320) -> (x+y=w341:i32)
              n117 = Add(x=w320, y=1) -> (x+y=→"HV Step":i32)
              n118 = flat-sequence {
                tunnel: w341 -> [w351]
                tunnel: w340 -> [w350]
                tunnel: w339 -> [w349]
                tunnel: w338 -> [w348]
                tunnel: [w347] -> w337
                tunnel: [w345] -> w336
                tunnel: [w345] -> w334
                tunnel: [w346] -> w333
                tunnel: [w344] -> w327
                tunnel: [w345] -> _
                tunnel: [w344] -> w326
                tunnel: w336 -> [w356]
                tunnel: [w356] -> w335
                tunnel: w334 -> [w355]
                tunnel: w333 -> [w354]
                tunnel: [w353] -> w328
                tunnel: w327 -> [w353]
                tunnel: w326 -> [w352]
                tunnel: [w352] -> w325
                tunnel: w335 -> [w359]
                tunnel: [w358] -> w329
                tunnel: w328 -> [w358]
                tunnel: w325 -> [w357]
                tunnel: [w357] -> w324
                tunnel: [w363] -> w330
                tunnel: w329 -> [w363]
                tunnel: w324 -> [w362]
                tunnel: [w362] -> w323
                tunnel: [w379] -> w331
                tunnel: w330 -> [w379]
                tunnel: w323 -> [_]
                tunnel: w322 -> [w377]
                tunnel: w322 -> [w381]
                tunnel: [w380] -> w332
                tunnel: w331 -> [w380]
                tunnel: w322 -> [w388]
                tunnel: w341 -> [w390]
                tunnel: w337 -> [w386]
                tunnel: w332 -> [w387]
                frame #0 {
                  n119 = call "HV_ReadHV.vi"("Run"=w351, "HV Channel"=w348, "DAQ Channel"=w349, "PMT"=w350) -> ("Voltages"=w346:string[], "DAQ Channel Out"=w344:string[], "HV Channel Out"=w345:string[], "PMT Out"=w347:string[])  [unwired: 4 in]
                }
                frame #1 {
                  # "Set voltages"
                  n120 = call "HV_VSet_Multi.vi"("Voltage"=w354, "Channel"=w355) -> ()  [unwired: 9 in, 1 out]
                }
                frame #2 {
                  n121 = for {
                    tunnel: w359 -> [w360] mode=indexing
                    # "Power on"
                    n122 = call "HV_Onstate_Single.vi"("On/Off"="On", "Channel"=w360) -> ()  [unwired: 9 in, 1 out]
                  }
                }
                frame #3 {
                  w365 = 1000 ("y")
                  w364 = 20
                  # "Wait"
                  n123 = Tick Count (ms)() -> (millisecond timer value=w366:u32)
                  n124 = Multiply(x=w364, y=w365) -> (x*y=w367:i32)
                  n125 = while {
                    tunnel: w366 -> [w373]
                    tunnel: w365 -> [w371]
                    tunnel: w364 -> [w370]
                    stop <- w369 stop-if-true
                    n126 = Tick Count (ms)() -> (millisecond timer value=w374:u32)
                    n127 = Subtract(x=w374, y=w373) -> (x-y=w372:u32)
                    n128 = Quotient & Remainder(x=w372, y=w371) -> (floor(x/y)=w368:u32)  [unwired: 1 out]
                    n129 = Greater?(x=w368, y=w370) -> (0:w369:bool)
                  }
                  n130 = Wait (ms)(milliseconds to wait=w367) -> ()  [unwired: 1 out]
                }
                frame #4 {
                  # "Clear files"
                  n131 = call <vilib>:"Application Directory.vi"() -> ("Application Directory"=w378:path)
                  n132 = Build Path(base path=w378, name or relative path=w377) -> (appended path=w376:path)
                  n133 = call <vilib>:"System Exec.vi"("working directory"=w376, "command line"="rm -f *.dat") -> ()  [unwired: 6 in, 4 out]
                }
                frame #5 {
                  w384 = "Gain.sh"  # Name of Bash Script
                  # "Run wavedump"
                  n134 = call <vilib>:"Application Directory.vi"() -> ("Application Directory"=w383:path)
                  n135 = Build Path(base path=w383, name or relative path=w381) -> (appended path=w382:path)
                  n136 = call "Send_Bash_Command.vi"("working directory"=w382, "Bash script"=w384) -> ()  [unwired: 4 in, 5 out]
                }
                frame #6 {
                  # "Move files"
                  n137 = Number To Decimal String(number=w390) -> (decimal integer string=w389:string)  [unwired: 1 in]
                  n138 = call "Move_Files_Gain.vi"("Folder name"="Folder name", "Run"=w389, "PMTs"=w386, "Channel"=w387, "Folder Containing Bash Script"=w388, "Name of Folder to\nCopy PMT File to"=w388) -> ()  [unwired: 6 in]
                }
              }
            }
          }
          frame #3 {
            n139 = for {
              tunnel: w395 -> [w396] mode=indexing
              # "Power on"
              n140 = call "HV_Onstate_Single.vi"("On/Off"="Off", "Channel"=w396) -> ()  [unwired: 9 in, 1 out]
            }
            n141 = call <vilib>:"Application Directory.vi"() -> ("Application Directory"=w394:path)
            n142 = Build Path(base path=w394, name or relative path="Gain") -> (appended path=w393:path)
            n143 = call <vilib>:"System Exec.vi"("working directory"=w393, "command line"="rm -f *.dat") -> ()  [unwired: 6 in, 4 out]
          }
        }
      }
      event Panel Close? {
        # "Send the 'Confirm Quit' message if the user closes the panel of the VI. Discard the event so the 'Confirm Quit' message has a chance to run."
        n144 = event-data() -> ()  [unwired: 1 in, 1 out]
        n145 = call-poly "Enqueue Message.vi"("Priority Message? (F)"=TRUE, "Message"="Confirm Quit", "Message Queue"=w402) -> ("error out"=w401:errorcluster, "dup Message Queue"=w400:refnum<queue>)  [unwired: 7 in]
        n146 = event-data("Discard?"=TRUE) -> ()  [unwired: 1 in, 1 out]
      }
      event Application Instance Close {
        # "Add switch HV off in here"
        # "#CodeRecommended - When a project closes, all VIs within that project are aborted and leave memory. However, any code placed in this event frame is guaranteed to run to completion, so add any cleanup code that absolutely must happen here."
        n147 = event-data() -> ()  [unwired: 1 in, 1 out]
        n148 = for {
          N: 18 -> [_]
          i -> [w407]
          # "Turn all channels off"
          n149 = Number To Decimal String(number=w407) -> (decimal integer string=w408:string)  [unwired: 1 in]
          n150 = call "HV_Onstate_Single.vi"("On/Off"="Off", "Channel"=w408) -> ()  [unwired: 9 in, 1 out]
        }
      }
      event "Exit": Value Change {
        n151 = event-data() -> ()  [unwired: 1 in, 1 out]
        n152 = for {
          N: 18 -> [_]
          i -> [w416]
          # "Turn all channels off"
          n153 = Number To Decimal String(number=w416) -> (decimal integer string=w417:string)  [unwired: 1 in]
          n154 = call "HV_Onstate_Single.vi"("On/Off"="Off", "Channel"=w417) -> ()  [unwired: 9 in, 1 out]
        }
        n155 = call-poly "Enqueue Message.vi"("Priority Message? (F)"=TRUE, "Message"="Exit", "Message Queue"=w414) -> ("error out"=w413:errorcluster, "dup Message Queue"=w412:refnum<queue>)  [unwired: 7 in]
      }
      event User Event {
        # "The Message Handling Loop processed an \"Exit\" message, which fired this event to stop the Event Handling Loop."
        n156 = event-data() -> ()  [unwired: 1 in, 1 out]
        n157 = local write "HV Control Readout"("\"Exit\" button pressed" ("VI Stopped")) -> ()
      }
    }
    n158 = call "Error Handler - Event Handling Loop.vi"("error in (no error)"=w46, "Message Queue"=w44) -> ("dup error in"=w43:errorcluster)  [unwired: 8 in, 1 out]
  }
  n159 = Merge Errors(w8, w18) -> (w7:errorcluster)
  n160 = while {
    tunnel: w4 -> [w425]
    shift-right: [w432] -> _
    shift-left: w3 -> [w433]
    tunnel: w6 -> [w430]
    tunnel: w7 -> [w429]
    tunnel: [w423] -> w16
    stop <- w431 stop-if-true
    # "HV Message Handling Loop"
    n161 = call "Dequeue Message.vi"("error in (no error)"=w429, "Message Queue"=w425) -> ("error out"=w428:errorcluster, "Message Data"=w426:variant, "Message"=w427:string, "dup Message Queue"=w424:refnum<queue>)  [unwired: 6 in]
    n162 = case "Message Cases" shown="\"Initialize\"" w427 {
      selector: w427 -> [_ _ _ _ _ _ _ _ _ _ _ w523]
      tunnel: w424 -> [w441 w451 w458 w465 w472 w479 w486 _ _ w507 w522 _]
      tunnel: w428 -> [w447 w453 w460 w467 w474 w481 w488 w495 w504 w511 w515 _]
      tunnel: [w448 w454 w461 w468 w475 w482 w489 w496 w498 w509 w518 w524] -> w422
      tunnel: w433 -> [w446 w455 w462 w469 w476 w483 w490 w497 w503 w510 w521 w525]
      tunnel: [w445 w455 w462 w469 w476 w483 w490 w497 w503 w510 w521 w525] -> w432
      tunnel: [_ _ _ _ _ _ _ _ _ _ TRUE _] -> w431
      tunnel: w426 -> [_ _ _ _ _ _ _ w494 w502 _ w512 _]
      tunnel: w430 -> [_ _ _ _ _ _ _ _ _ _ w517 _]
      frame "Initialize" {
        w440 = "PMT Test Control" ("Initial Message")
        # "bundle by name"
        # "Bundle control references and a sample string value."
        # "Initialize - All initialization work should take place in this message, since other loops can potentially enqueue messages that execute immediately after this one."
        n163 = control-ref of="HV Control Readout"() -> (w444:refnum<vi>)
        n164 = control-ref of="VMax"() -> (w438:refnum<vi>)
        n165 = control-ref of="ISet"() -> (w437:refnum<vi>)
        n166 = control-ref of="power"() -> (w439:refnum<vi>)
        n167 = control-ref of="Off"() -> (w434:refnum<vi>)
        n168 = control-ref of="VSet"() -> (w436:refnum<vi>)
        n169 = control-ref of="Ramp"() -> (w435:refnum<vi>)
        n170 = control-ref of="Exit"() -> (w443:refnum<vi>)
        n171 = call-poly "Enqueue Message.vi"("error in (no error)"=w447, "Message Data"=w440, "Message"="Update Display", "Message Queue"=w441) -> ("error out"=w448:errorcluster)  [unwired: 6 in, 1 out]
        n172 = Bundle By Name(cluster=w446, "VMax Ref"=w438, "ISet Ref"=w437, "power Ref"=w439, "Off Ref"=w434, "VSet Ref"=w436, "Ramp Ref"=w435, "Data Display Ref"=w444, "Exit Button Ref"=w443, "String"=w440) -> (w445:T3)
      }
      frame "power" {
        # "Send string to \"Update Display\" message"
        # "#CodeNeeded - Perform whatever actions correspond to the \"Something Else\" message."
        # "Something Else - Replace this message with functionality for your own application."
        n173 = call-poly "Enqueue Message.vi"("error in (no error)"=w453, "Message Data"="Setting power" ("\"Do Something Else\" button pressed"), "Message"="Update Display", "Message Queue"=w451) -> ("error out"=w452:errorcluster)  [unwired: 6 in, 1 out]
        n174 = Merge Errors(w452) -> (w454:errorcluster)
      }
      frame "ISet" {
        # "Send string to \"Update Display\" message"
        # "#CodeNeeded - Perform whatever actions correspond to the \"Something Else\" message."
        # "Something Else - Replace this message with functionality for your own application."
        n175 = call-poly "Enqueue Message.vi"("error in (no error)"=w460, "Message Data"="Setting current" ("\"Do Something Else\" button pressed"), "Message"="Update Display", "Message Queue"=w458) -> ("error out"=w459:errorcluster)  [unwired: 6 in, 1 out]
        n176 = Merge Errors(w459) -> (w461:errorcluster)
      }
      frame "VSet" {
        # "Send string to \"Update Display\" message"
        # "#CodeNeeded - Perform whatever actions correspond to the \"Something Else\" message."
        # "Something Else - Replace this message with functionality for your own application."
        n177 = call-poly "Enqueue Message.vi"("error in (no error)"=w467, "Message Data"="Setting voltage" ("\"Do Something Else\" button pressed"), "Message"="Update Display", "Message Queue"=w465) -> ("error out"=w466:errorcluster)  [unwired: 6 in, 1 out]
        n178 = Merge Errors(w466) -> (w468:errorcluster)
      }
      frame "VMax" {
        # "Send string to \"Update Display\" message"
        # "#CodeNeeded - Perform whatever actions correspond to the \"Something Else\" message."
        # "Something Else - Replace this message with functionality for your own application."
        n179 = call-poly "Enqueue Message.vi"("error in (no error)"=w474, "Message Data"="Setting max voltage" ("\"Do Something Else\" button pressed"), "Message"="Update Display", "Message Queue"=w472) -> ("error out"=w473:errorcluster)  [unwired: 6 in, 1 out]
        n180 = Merge Errors(w473) -> (w475:errorcluster)
      }
      frame "Ramp" {
        # "Send string to \"Update Display\" message"
        # "#CodeNeeded - Perform whatever actions correspond to the \"Something Else\" message."
        # "Something Else - Replace this message with functionality for your own application."
        n181 = call-poly "Enqueue Message.vi"("error in (no error)"=w481, "Message Data"="Setting ramp rates" ("\"Do Something Else\" button pressed"), "Message"="Update Display", "Message Queue"=w479) -> ("error out"=w480:errorcluster)  [unwired: 6 in, 1 out]
        n182 = Merge Errors(w480) -> (w482:errorcluster)
      }
      frame "Off" {
        # "Send string to \"Update Display\" message"
        # "#CodeNeeded - Perform whatever actions correspond to the \"Something Else\" message."
        # "Something Else - Replace this message with functionality for your own application."
        n183 = call-poly "Enqueue Message.vi"("error in (no error)"=w488, "Message Data"="Turning HV off" ("\"Do Something Else\" button pressed"), "Message"="Update Display", "Message Queue"=w486) -> ("error out"=w487:errorcluster)  [unwired: 6 in, 1 out]
        n184 = Merge Errors(w487) -> (w489:errorcluster)
      }
      frame "Update Display" {
        # "#CodeRecommended - If you wish to decouple the Message Handling Loop from your user interface, consider creating User Events (like the \"Stop\" event in this VI) to message the Event Handling Loop whenever the user interface needs updating."
        # "Update Display - Convert the message data to a string to display in the Data Display indicator."
        n185 = Variant To Data(error in=w495, type="", Variant=w494) -> (data=→"HV Control Readout":string, error out=w492:errorcluster)
        n186 = Merge Errors(w492) -> (w496:errorcluster)
      }
      frame "Error" {
        # "#CodeRecommended - If you ever change the name of this \"Error\" message, you'll need to update the name in the Check Loop Error.vi as well."
        # "#CodeRecommended - Consider creating a system for logging errors in some way. These errors are for notification purposes only. Handling of specific errors should be performed in the message frames that generated the error."
        # "Error - Display an error dialog. This message is sent by the \"Error Handler\" VIs at the end of other loops in this application."
        n187 = Variant To Data(error in=w504, type=errorcluster {"status"=FALSE, "code"=0, "source"=""} ("error constant"), Variant=w502) -> (data=w500:errorcluster, error out=w499:errorcluster)
        n188 = call <vilib>:"Simple Error Handler.vi"("error in (no error)"=w500) -> ()  [unwired: 4 in, 5 out]
        n189 = Merge Errors(w499) -> (w498:errorcluster)
      }
      frame "Confirm Quit" {
        # "#CodeNeeded - If you want to provide an \"Are you sure\" dialog (or some other notification) before the application exits, place that code here. This message is typically sent from a Panel Close? event."
        # "Confirm Quit - Message that can confirm whether or not the user wants to exit the application."
        n190 = call-poly "Enqueue Message.vi"("Priority Message? (F)"=TRUE, "error in (no error)"=w511, "Message"="Exit", "Message Queue"=w507) -> ("error out"=w508:errorcluster)  [unwired: 6 in, 1 out]
        n191 = Merge Errors(w508) -> (w509:errorcluster)
      }
      frame "Exit" {
        # "Stop the VI"
        # "Release the message queue reference"
        # "#CodeNeeded - Add any required cleanup code here. Note that if 'Exit' was called as a result of an error, an error dialog will be displayed. Add any custom error handling for an 'Exit' condition here as well."
        # "Exit - Exit the application."
        n192 = Release Queue(queue=w522, error in (no error)=w515) -> (error out=w519:errorcluster)  [unwired: 1 in, 2 out]
        n193 = Variant To Data(type=errorcluster {"status"=FALSE, "code"=0, "source"=""} ("error constant"), Variant=w512) -> (data=w513:errorcluster)  [unwired: 1 in, 1 out]
        n194 = call <vilib>:"Simple Error Handler.vi"("error in (no error)"=w513) -> ()  [unwired: 4 in, 5 out]
        n195 = call "Fire User Event - Stop.vi"("User Event - Stop"=w517) -> ("error out"=w516:errorcluster)  [unwired: 10 in]
        n196 = Merge Errors(w516, w519) -> (w518:errorcluster)
      }
      frame Default {
        # "'Default' case only runs if there is a message that isn't defined in any of the other cases.  Output a programming error."
        n197 = xnode "Error Ring"("parameter 0"=w523) -> ("error out"=w524:errorcluster)
      }
    }
    n198 = call "Error Handler - Message Handling Loop.vi"("error in (no error)"=w422, "Message Queue"=w424) -> ("dup error in"=w423:errorcluster)  [unwired: 8 in, 1 out]
  }
  n199 = while {
    tunnel: w1 -> [w536]
    shift-right: [w543] -> _
    shift-left: w2 -> [w544]
    tunnel: w6 -> [w541]
    tunnel: w7 -> [w540]
    tunnel: [w534] -> w5
    stop <- w542 stop-if-true
    # "Wavedump Message Handling Loop"
    n200 = call "Dequeue Message.vi"("error in (no error)"=w540, "Message Queue"=w536) -> ("error out"=w539:errorcluster, "Message Data"=w537:variant, "Message"=w538:string, "dup Message Queue"=w535:refnum<queue>)  [unwired: 6 in]
    n201 = case "Message Cases" shown="\"Initialize\"" w538 {
      selector: w538 -> [_ _ _ _ _ _ _ _ _ _ w622]
      tunnel: w535 -> [w548 _ _ w571 w579 w586 w593 w600 w607 w621 _]
      tunnel: w539 -> [w553 w559 w568 w575 w578 w585 w592 w599 w606 w614 _]
      tunnel: [w554 w560 w562 w573 w581 w588 w595 w602 w609 w617 w623] -> w533
      tunnel: w544 -> [w552 w561 w567 w574 w582 w589 w596 w603 w610 w620 w624]
      tunnel: [w551 w561 w567 w574 w582 w589 w596 w603 w610 w620 w624] -> w543
      tunnel: [_ _ _ _ _ _ _ _ _ TRUE _] -> w542
      tunnel: w537 -> [_ w558 w566 _ _ _ _ _ _ w611 _]
      tunnel: w541 -> [_ _ _ _ _ _ _ _ _ w616 _]
      frame "Initialize" {
        w547 = "PMT Test Control" ("Initial Message")
        # "bundle by name"
        # "Bundle control references and a sample string value."
        # "Initialize - All initialization work should take place in this message, since other loops can potentially enqueue messages that execute immediately after this one."
        n202 = control-ref of="Test Control Readout"() -> (w550:refnum<vi>)
        n203 = control-ref of="Exit"() -> (w546:refnum<vi>)
        n204 = control-ref of="wavedump"() -> (w545:refnum<vi>)
        n205 = call-poly "Enqueue Message.vi"("error in (no error)"=w553, "Message Data"=w547, "Message"="Update Display", "Message Queue"=w548) -> ("error out"=w554:errorcluster)  [unwired: 6 in, 1 out]
        n206 = Bundle By Name(cluster=w552, "wavedump Ref"=w545, "Data Display Ref"=w550, "Exit Button Ref"=w546, "String"=w547) -> (w551:T2)
      }
      frame "Update Display" {
        # "#CodeRecommended - If you wish to decouple the Message Handling Loop from your user interface, consider creating User Events (like the \"Stop\" event in this VI) to message the Event Handling Loop whenever the user interface needs updating."
        # "Update Display - Convert the message data to a string to display in the Data Display indicator."
        n207 = Variant To Data(error in=w559, type="", Variant=w558) -> (data=→"Test Control Readout":string, error out=w556:errorcluster)
        n208 = Merge Errors(w556) -> (w560:errorcluster)
      }
      frame "Error" {
        # "#CodeRecommended - If you ever change the name of this \"Error\" message, you'll need to update the name in the Check Loop Error.vi as well."
        # "#CodeRecommended - Consider creating a system for logging errors in some way. These errors are for notification purposes only. Handling of specific errors should be performed in the message frames that generated the error."
        # "Error - Display an error dialog. This message is sent by the \"Error Handler\" VIs at the end of other loops in this application."
        n209 = Variant To Data(error in=w568, type=errorcluster {"status"=FALSE, "code"=0, "source"=""} ("error constant"), Variant=w566) -> (data=w564:errorcluster, error out=w563:errorcluster)
        n210 = call <vilib>:"Simple Error Handler.vi"("error in (no error)"=w564) -> ()  [unwired: 4 in, 5 out]
        n211 = Merge Errors(w563) -> (w562:errorcluster)
      }
      frame "Confirm Quit" {
        # "#CodeNeeded - If you want to provide an \"Are you sure\" dialog (or some other notification) before the application exits, place that code here. This message is typically sent from a Panel Close? event."
        # "Confirm Quit - Message that can confirm whether or not the user wants to exit the application."
        n212 = call-poly "Enqueue Message.vi"("Priority Message? (F)"=TRUE, "error in (no error)"=w575, "Message"="Exit", "Message Queue"=w571) -> ("error out"=w572:errorcluster)  [unwired: 6 in, 1 out]
        n213 = Merge Errors(w572) -> (w573:errorcluster)
      }
      frame "wavedump" {
        # "#CodeNeeded - If you want to provide an \"Are you sure\" dialog (or some other notification) before the application exits, place that code here. This message is typically sent from a Panel Close? event."
        # "Confirm Quit - Message that can confirm whether or not the user wants to exit the application."
        n214 = call-poly "Enqueue Message.vi"("error in (no error)"=w578, "Message Data"="Powering up channels, please wait 20 seconds", "Message"="Update Display", "Message Queue"=w579) -> ("error out"=w580:errorcluster)  [unwired: 6 in, 1 out]
        n215 = Merge Errors(w580) -> (w581:errorcluster)
      }
      frame "Power On" {
        # "#CodeNeeded - If you want to provide an \"Are you sure\" dialog (or some other notification) before the application exits, place that code here. This message is typically sent from a Panel Close? event."
        # "Confirm Quit - Message that can confirm whether or not the user wants to exit the application."
        n216 = call-poly "Enqueue Message.vi"("error in (no error)"=w585, "Message Data"="Writing script", "Message"="Update Display", "Message Queue"=w586) -> ("error out"=w587:errorcluster)  [unwired: 6 in, 1 out]
        n217 = Merge Errors(w587) -> (w588:errorcluster)
      }
      frame "bash written" {
        # "#CodeNeeded - If you want to provide an \"Are you sure\" dialog (or some other notification) before the application exits, place that code here. This message is typically sent from a Panel Close? event."
        # "Confirm Quit - Message that can confirm whether or not the user wants to exit the application."
        n218 = call-poly "Enqueue Message.vi"("error in (no error)"=w592, "Message Data"="Clearing old files", "Message"="Update Display", "Message Queue"=w593) -> ("error out"=w594:errorcluster)  [unwired: 6 in, 1 out]
        n219 = Merge Errors(w594) -> (w595:errorcluster)
      }
      frame "files cleared" {
        # "#CodeNeeded - If you want to provide an \"Are you sure\" dialog (or some other notification) before the application exits, place that code here. This message is typically sent from a Panel Close? event."
        # "Confirm Quit - Message that can confirm whether or not the user wants to exit the application."
        n220 = call-poly "Enqueue Message.vi"("error in (no error)"=w599, "Message Data"="Running wavedump", "Message"="Update Display", "Message Queue"=w600) -> ("error out"=w601:errorcluster)  [unwired: 6 in, 1 out]
        n221 = Merge Errors(w601) -> (w602:errorcluster)
      }
      frame "wavedump finished" {
        # "#CodeNeeded - If you want to provide an \"Are you sure\" dialog (or some other notification) before the application exits, place that code here. This message is typically sent from a Panel Close? event."
        # "Confirm Quit - Message that can confirm whether or not the user wants to exit the application."
        n222 = call-poly "Enqueue Message.vi"("error in (no error)"=w606, "Message Data"="Wavedump finished", "Message"="Update Display", "Message Queue"=w607) -> ("error out"=w608:errorcluster)  [unwired: 6 in, 1 out]
        n223 = Merge Errors(w608) -> (w609:errorcluster)
      }
      frame "Exit" {
        # "Need a proper exit condition"
        # "Stop the VI"
        # "Release the message queue reference"
        # "#CodeNeeded - Add any required cleanup code here. Note that if 'Exit' was called as a result of an error, an error dialog will be displayed. Add any custom error handling for an 'Exit' condition here as well."
        # "Exit - Exit the application."
        n224 = Release Queue(queue=w621, error in (no error)=w614) -> (error out=w618:errorcluster)  [unwired: 1 in, 2 out]
        n225 = Variant To Data(type=errorcluster {"status"=FALSE, "code"=0, "source"=""} ("error constant"), Variant=w611) -> (data=w612:errorcluster)  [unwired: 1 in, 1 out]
        n226 = call <vilib>:"Simple Error Handler.vi"("error in (no error)"=w612) -> ()  [unwired: 4 in, 5 out]
        n227 = call "Fire User Event - Stop.vi"("User Event - Stop"=w616) -> ("error out"=w615:errorcluster)  [unwired: 10 in]
        n228 = Merge Errors(w615, w618) -> (w617:errorcluster)
      }
      frame Default {
        # "'Default' case only runs if there is a message that isn't defined in any of the other cases.  Output a programming error."
        n229 = xnode "Error Ring"("parameter 0"=w622) -> ("error out"=w623:errorcluster)
      }
    }
    n230 = call "Error Handler - Message Handling Loop.vi"("error in (no error)"=w533, "Message Queue"=w535) -> ("dup error in"=w534:errorcluster)  [unwired: 8 in, 1 out]
  }
  n231 = Unregister For Events(event registration refnum=w12, error in=w10) -> (error out=w13:errorcluster)
  n232 = Merge Errors "Merge Errors"(w13, w16, w5) -> (w14:errorcluster)
  n233 = call "Destroy User Event - Stop.vi"("error in (no error)"=w14, "User Event - Stop"=w6) -> ("error out"=w11:errorcluster)  [unwired: 9 in]
  n234 = disable-structure shown="RUN_TIME_ENGINE==True" {
    disable-tunnel: w11 -> [_ _]
    frame condition #0 (active) {
    }
    frame condition #1 {
      # "Call Quit LabVIEW if running as a built application."
      n235 = Quit LabVIEW() -> ()  [unwired: 1 in]
    }
  }
